vi "04. Downloader.vi"(8 "error in":errorcluster) -> (0 "error out":errorcluster)   [LabVIEW 2019]
panel:
  out "Numeric":i32
  out "Array":dbl[](array[numeric])
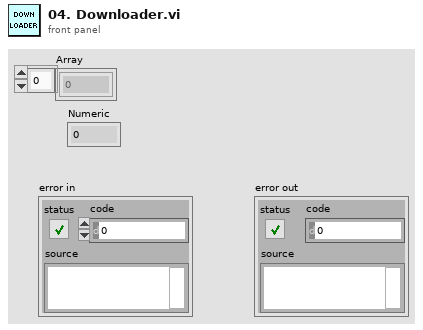
[diagram p1: front panel]
types:
  T1 = enum16{"Standard", "Buffered", "CRLF", "Immediate"}
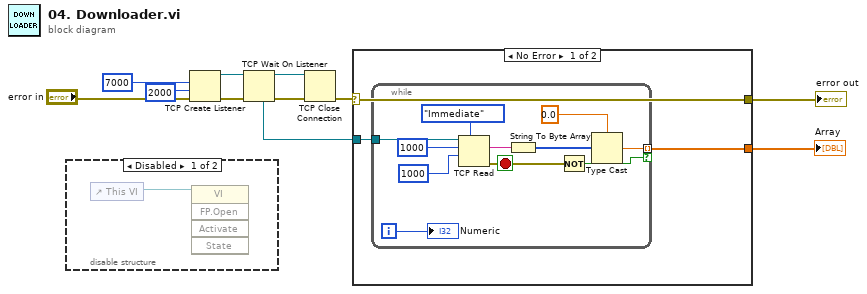
[diagram p0: block diagram]
diagram:
  n1 = disable-structure shown="Disabled" {
    frame Disabled {
      n2 = control-ref of="This VI"() -> (w12:refnum<vi>)
      n3 = invoke class="VI" method="FP.Open"(reference=w12) -> ()  [unwired: 4 in, 5 out]
    }
    frame Enabled {
    }
  }
  n4 = TCP Create Listener(8:"error in", 9:2000 ("timeout ms (25000)"), 10:u16 7000 ("port")) -> (0:w6:errorcluster, 3:w8:refnum<k5>)  [unwired: 2 in, 1 out]
  n5 = TCP Wait On Listener(8:w6, 11:w8) -> (0:w5:errorcluster, 3:w7:refnum<k5>, 4:w4:refnum<k5>)  [unwired: 2 in, 2 out]
  n6 = TCP Close Connection(connection ID=w7, error in (no error)=w5) -> (error out=w3:errorcluster)  [unwired: 1 in, 1 out]
  n7 = case shown="No Error" w3 {
    selector: w3 -> [w13 w27]
    tunnel: w4 -> [w15 _]
    tunnel: [w13 w27] -> w2
    tunnel: [w14 _] -> w1
    frame No Error {
      n8 = while {
        tunnel: w15 -> [w26]
        tunnel: [w17] -> w14 mode=indexing if=w16
        i -> [w21]
        stop <- w20 stop-if-true
        n9 = TCP Read(connection ID=w26, bytes to read=1000, 7:T1."Immediate" ("mode (standard)"), 9:1000 ("timeout ms (25000)")) -> (data out=w22:string, error out=w20:errorcluster)  [unwired: 1 in, 1 out]
        n10 = String To Byte Array(string=w22) -> (unsigned byte array=w19:u8[])
        n11 = Not(x=w20) -> (.not. x?=w16:bool)
        n12 = Type Cast(type=0.0, x=w19) -> (*(type *) &x=w17:dbl)
        "Numeric" <- w21
      }
    }
    frame Error {
    }
  }
  "error out" <- w2
  "Array" <- w1
